vi "Send To Caller.vi"(8 "error in (no error)":errorcluster, 9 "Message Priority (Normal)":T1=enum."Normal", 10 "Actor in":refnum<class "Actor.lvclass">, 11 "Publisher Msg in":refnum<class "Publisher Msg.lvclass">) -> (0 "error out":errorcluster, 1 "Msg Dropped?":bool, 2 "Actor out":refnum<class "Actor.lvclass">)   [LabVIEW 2020, in "Publisher.lvlib" / "Publisher Msg.lvclass"]
doc: "Forward the Publisher Msg to the Publisher with the given Message Priority."
uses:
  Publisher Msg.lvclass
  PPL/HDH.Actor Framework.Core.Actor.lvlibp/1abvi3w/vi.lib/ActorFramework/Actor/Actor.lvclass
  PPL/HDH.Actor Framework.Core.Actor.lvlibp/1abvi3w/vi.lib/ActorFramework/Message Enqueuer/Message Priority.ctl
  Publisher Msg.lvclass/Publisher Msg.ctl
  Read Message Priority.vi
  PPL/HDH.Actor Framework.Core.Actor.lvlibp/1abvi3w/vi.lib/ActorFramework/Actor/Read Caller Enqueuer.vi
  PPL/HDH.Actor Framework.Core.Actor.lvlibp/1abvi3w/vi.lib/ActorFramework/Message Enqueuer/Enqueue.vi
  Publisher/Publisher.lvclass
  PPL/HDH.Actor Framework.Core.Utility.lvlibp
  PPL/HDH.Actor Framework.Core.Actor.lvlibp/1abvi3w/vi.lib/ActorFramework/Message Enqueuer/Message Enqueuer.lvclass
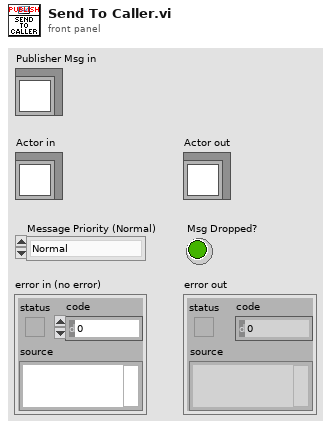
[diagram p1: front panel]
types:
  T1 = typedef "HDH.Actor Framework.Core.Actor.lvlibp/Message Enqueuer.lvclass/Message Priority.ctl" = enum16{"Low", "Normal", "High"}
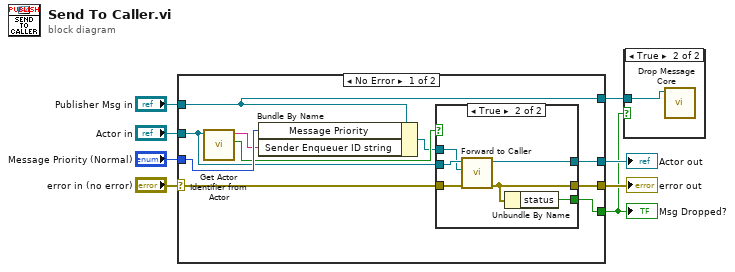
[diagram p0: block diagram]
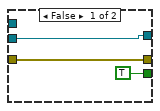
[diagram p3: hidden frame]
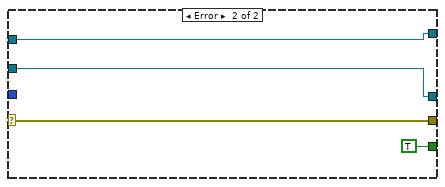
[diagram p4: hidden frame]
diagram:
  n1 = case shown="No Error" "error in (no error)" {
    selector: "error in (no error)" -> [w12 w31]
    tunnel: [w11 w31] -> w7
    tunnel: "Publisher Msg in" -> [w9 w28]
    tunnel: [w13 w30] -> w5
    tunnel: "Actor in" -> [w14 w30]
    tunnel: "Message Priority (Normal)" -> [w18 _]
    tunnel: [w10 TRUE] -> w2
    tunnel: [w9 w28] -> w1
    frame No Error {
      n2 = call "Get Actor Identifier from Actor.vi"("Actor in"=w14) -> ("Valid Enqueuer?"=w16:bool, "Actor ID string out"=w17:string)  [unwired: 9 in]
      n3 = Bundle By Name(cluster=w9, "Message Priority"=w18, "Sender Enqueuer ID string"=w17) -> (w15:refnum<class "Publisher Msg.lvclass">)
      n4 = case shown="True" w16 {
        tunnel: w15 -> [_ w25]
        tunnel: w14 -> [w20 w27]
        tunnel: [w20 w26] -> w13
        tunnel: w12 -> [w21 w24]
        tunnel: [w21 w23] -> w11
        tunnel: [TRUE w22] -> w10
        frame False {
        }
        frame True {
          n5 = call "Forward to Caller.vi"("error in (no error)"=w24, "Publisher Message"=w25, "Actor in"=w27) -> ("error out"=w23:errorcluster, "Actor out"=w26:refnum<class "Actor.lvclass">)  [unwired: 7 in]
          n6 = Unbundle By Name(w23) -> ("status"=w22:bool)
        }
      }
    }
    frame Error {
    }
  }
  "error out" <- w7
  "Actor out" <- w5
  "Msg Dropped?" <- w2
  n7 = case shown="True" w2 {
    tunnel: w1 -> [_ w32]
    frame False {
    }
    frame True {
      n8 = call-dynamic "Drop Message Core.vi"("Message in"=w32) -> ()  [unwired: 11 in]
    }
  }
